vi "Registerkartenverwaltung.vi"(8 "Fehler (Eingang, kein Fehler)":errorcluster, 9 "Sprachauswahl":u32, 10 "all rows":string[][](array[string]), 11 "Seiten":refnum<vi>[](array[refnum])) -> (0 "error out":errorcluster)   [LabVIEW 2020, in "Sprachverwaltung.lvlib"]
uses:
  Sprachverwaltung.lvlib
panel:
  out "Seiten out":refnum<vi>[](array[refnum])
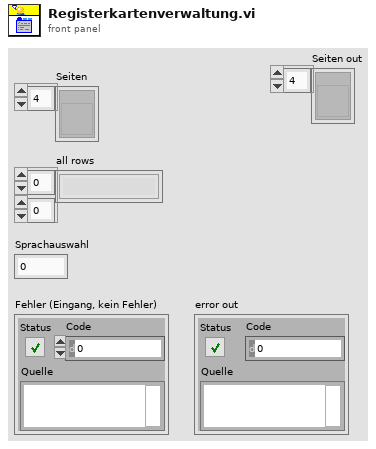
[diagram p1: front panel]
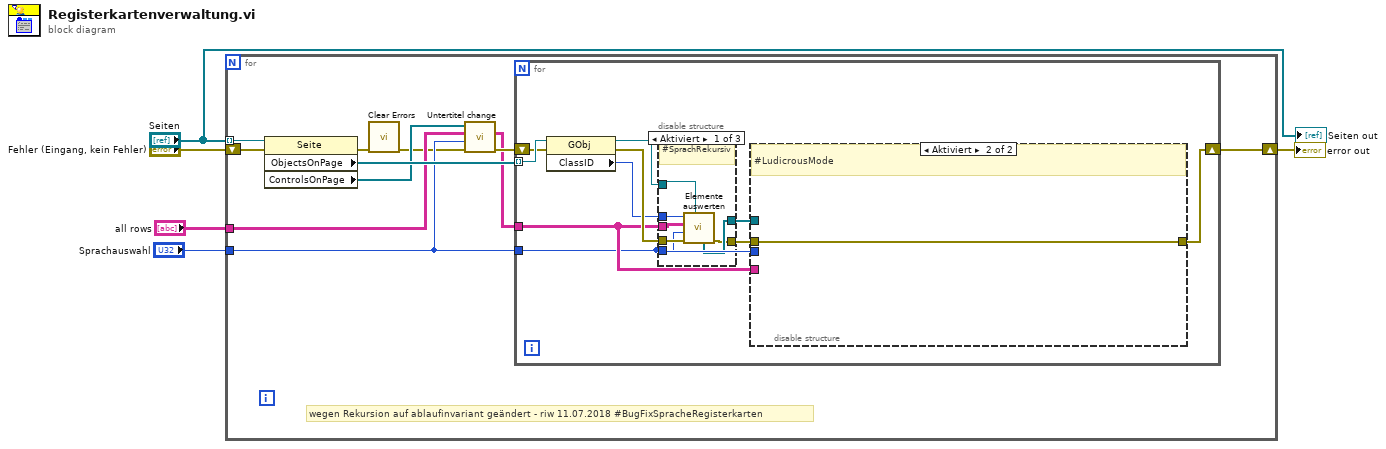
[diagram p0: block diagram]
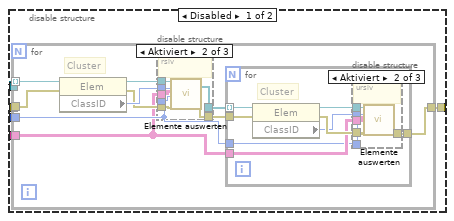
[diagram p2: hidden frame]
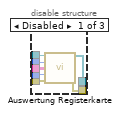
[diagram p3: hidden frame]
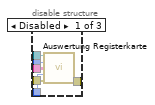
[diagram p5: hidden frame]
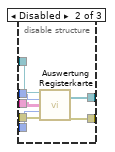
[diagram p7: hidden frame]
diagram:
  n1 = for {
    tunnel: "Seiten" -> [w16] mode=indexing
    tunnel: "Sprachauswahl" -> [w12]
    tunnel: "all rows" -> [w13]
    shift-right: [w8] -> w1
    shift-left: "Fehler (Eingang, kein Fehler)" -> [w10]
    # "wegen Rekursion auf ablaufinvariant geändert - riw 11.07.2018 #BugFixSpracheRegisterkarten"
    n2 = property class="Seite"(reference=w16, error in=w10) -> (error out=w11:errorcluster, "ObjectsOnPage"=w15:refnum<vi>[], "ControlsOnPage"=w14:refnum<vi>[])  [unwired: 1 out]
    n3 = call <vilib>:"Clear Errors.vi"("error in (no error)"=w11) -> ("error out"=w6:errorcluster)  [unwired: 5 in, 1 out]
    n4 = call "Untertitel change.vi"("Fehler (Eingang, kein Fehler)"=w6, "Sprachauswahl"=w12, "Sprachdatei"=w13, "Controls[]"=w14) -> ("Fehler (Ausgang, kein Fehler)"=w9:errorcluster, "Sprachdatei out"=w7:string[][])  [unwired: 5 in, 1 out]
    n5 = for {
      tunnel: w15 -> [w26] mode=indexing
      tunnel: w12 -> [w19]
      tunnel: w7 -> [w20]
      shift-right: [w17] -> w8
      shift-left: w9 -> [w25]
      n6 = property class="GObj"(reference=w26, error in=w25) -> (reference out=w24:refnum<vi>, error out=w23:errorcluster, "ClassID"=w22:u32)
      n7 = disable-structure shown="Aktiviert" {
        disable-tunnel: w24 -> [w76 w89 _]
        disable-tunnel: w23 -> [w82 w88 _]
        disable-tunnel: w22 -> [w77 w87 _]
        disable-tunnel: [w81 w86 _] -> w21
        disable-tunnel: w20 -> [w80 w85 _]
        disable-tunnel: w19 -> [w79 w84 _]
        disable-tunnel: [w78 w83 _] -> w18
        frame Enabled {
          # "#SprachRekursiv"
          n8 = call "Elemente auswerten.vi"("GObject (Eingang)"=w76, "Fehler (Eingang, kein Fehler)"=w82, "Sprachauswahl"=w79, "all rows"=w80, "ClassID"=w77) -> ("error out"=w78:errorcluster, "Cluster Elemente[]"=w81:refnum<vi>[])  [unwired: 1 in, 4 out]
        }
        frame Disabled {
          n9 = call "Auswertung Registerkarte.vi"("GObject (Eingang)"=w89, "ClassID"=w87, "all rows"=w85, "Sprachauswahl"=w84, "Fehler (Eingang, kein Fehler)"=w88) -> ("Clusterelemente"=w86:refnum<vi>[], "error out"=w83:errorcluster)  [unwired: 9 in]
        }
        frame Disabled {
        }
      }
      n10 = disable-structure shown="Aktiviert" {
        disable-tunnel: w21 -> [w31 _]
        disable-tunnel: w20 -> [w30 _]
        disable-tunnel: w19 -> [w29 _]
        disable-tunnel: w18 -> [w28 w75]
        disable-tunnel: [w27 w75] -> w17
        frame Disabled {
          n11 = for {
            tunnel: w31 -> [w41] mode=indexing
            tunnel: w30 -> [w33]
            tunnel: w29 -> [w34]
            tunnel: w28 -> [w37]
            tunnel: [w32] -> w27
            # "Cluster"
            n12 = property class="Elem"(reference=w41, error in=w37) -> (reference out=w40:refnum<vi>, error out=w38:errorcluster, "ClassID"=w39:u32)
            n13 = disable-structure shown="Aktiviert" {
              disable-tunnel: w40 -> [w48 w55 _]
              disable-tunnel: w39 -> [w47 w54 _]
              disable-tunnel: w38 -> [w46 w53 _]
              disable-tunnel: [w45 w52 _] -> w36
              disable-tunnel: [w44 w51 _] -> w35
              disable-tunnel: w34 -> [w43 w50 _]
              disable-tunnel: w33 -> [w42 w49 _]
              frame Disabled {
                n14 = call "Auswertung Registerkarte.vi"("GObject (Eingang)"=w48, "ClassID"=w47, "all rows"=w42, "Sprachauswahl"=w43, "Fehler (Eingang, kein Fehler)"=w46) -> ("Clusterelemente"=w45:refnum<vi>[], "error out"=w44:errorcluster)  [unwired: 9 in]
              }
              frame Enabled {
                # "#SprachRekursiv"
                n15 = call "Elemente auswerten.vi"("GObject (Eingang)"=w55, "all rows"=w49, "Sprachauswahl"=w50, "Fehler (Eingang, kein Fehler)"=w53, "ClassID"=w54) -> ("Cluster Elemente[]"=w52:refnum<vi>[], "error out"=w51:errorcluster)  [unwired: 12 in, 1 out]
              }
              frame Disabled {
              }
            }
            n16 = for {
              tunnel: w36 -> [w60] mode=indexing
              tunnel: w35 -> [w59]
              tunnel: w34 -> [w57]
              tunnel: w33 -> [w58]
              tunnel: [w56] -> w32
              # "Cluster"
              n17 = property class="Elem"(reference=w60, error in=w59) -> (reference out=w61:refnum<vi>, error out=w63:errorcluster, "ClassID"=w62:u32)
              n18 = disable-structure shown="Aktiviert" {
                disable-tunnel: w63 -> [w68 w74 _]
                disable-tunnel: w62 -> [w67 w73 _]
                disable-tunnel: w61 -> [w66 w72 _]
                disable-tunnel: w58 -> [w65 w71 _]
                disable-tunnel: w57 -> [w64 w70 _]
                disable-tunnel: [_ w69 _] -> w56
                frame Disabled {
                  n19 = call "Auswertung Registerkarte.vi"("GObject (Eingang)"=w66, "ClassID"=w67, "all rows"=w65, "Sprachauswahl"=w64, "Fehler (Eingang, kein Fehler)"=w68) -> ()  [unwired: 9 in, 2 out]
                }
                frame Enabled {
                  # "#SprachRekursiv"
                  n20 = call "Elemente auswerten.vi"("GObject (Eingang)"=w72, "all rows"=w71, "Sprachauswahl"=w70, "Fehler (Eingang, kein Fehler)"=w74, "ClassID"=w73) -> ("error out"=w69:errorcluster)  [unwired: 12 in, 2 out]
                }
                frame Disabled {
                }
              }
            }
          }
        }
        frame Enabled {
          # "#LudicrousMode"
        }
      }
    }
  }
  "error out" <- w1
  "Seiten out" <- "Seiten"
